vi "Read Acquisition Time.vi"(8 "error in (no error)":errorcluster, 11 "VI Probe in":refnum<class "PL MKS VI Probe.lvclass">) -> (0 "error out":errorcluster, 2 "acquisition time, ms":u16(ring) items=["4.08", "6.08", "12.20", "20.96", "42.61", "85.20", "170.40", "348.60", "687.20"], 3 "VI Probe out":refnum<class "PL MKS VI Probe.lvclass">)   [LabVIEW 2015, in "PL MKS VI Probe.lvclass"]
doc: "Reads acquisition time."
uses:
  PL MKS VI Probe.lvclass
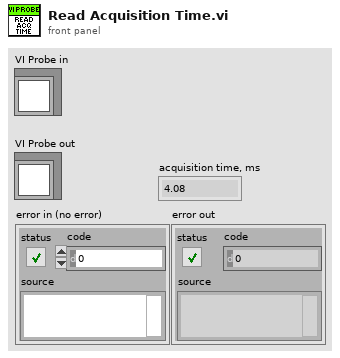
[diagram p1: front panel]
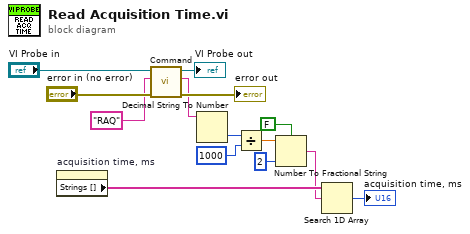
[diagram p0: block diagram]
diagram:
  n1 = property on="acquisition time, ms" class="Ring (strict)"() -> ("Strings []"=w4:string[])  [unwired: 2 in, 2 out]
  n2 = call "Command.vi"("error in (no error)"="error in (no error)", "command"="RAQ" ("format string"), "VI Probe in"="VI Probe in") -> ("error out"=→"error out":errorcluster, "response data"=w9:string, "VI Probe out"=→"VI Probe out":refnum<class "PL MKS VI Probe.lvclass">)  [unwired: 6 in]
  n3 = Decimal String To Number(string=w9) -> (number=w8:i32)  [unwired: 2 in, 1 out]
  n4 = Divide(x=w8, y=1000) -> (x/y=w7:dbl)
  n5 = Number To Fractional String(use system decimal point (T)=FALSE, number=w7, precision (6)=i16 2) -> (F-format string=w3:string)  [unwired: 1 in]
  n6 = Search 1D Array(1D array=w4, element=w3) -> (index of element=→"acquisition time, ms":i32)  [unwired: 1 in]
